vi "add.vi"(11 "LabVIEW Web Service Request":refnum<class "Web Request.lvclass">) -> ()   [LabVIEW 2014]
doc: "/lvwd-components-start/calc/add endpoint.\n\nExpects a JSON POST HTTP Request with a body containing a JSON object similar to the following:\n{ \"first\": \"5\", \"second\": \"6\" }\n\nA valid request returns a JSON object similar to the following:\n{\"sum\": 11}\n\nAn invalid request that is handelable returns HTTP Status Code 500 and a JSON object similar to:\n{\n \"message\": \"invalid parameters\",\n \"error\": {\n \"status\": true,\n \"code\": 5001,\n \"source\": \"notsoawesome.vi\",\n }\n}\n\nAn invalid request that cannot be handled MAY return an error code other than 200 and a response other than JSON (such as HTML, XML, etc)"
uses:
  <vilib>/wsapi/Web Request.lvclass
  Web Resources SubVIs/lvwd-components-start-calc.lvlib
  Utilities/lvwd-components-start-utilities.lvlib
panel:
  out "Error Out":errorcluster
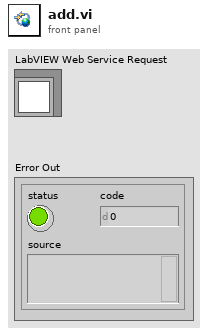
[diagram p1: front panel]
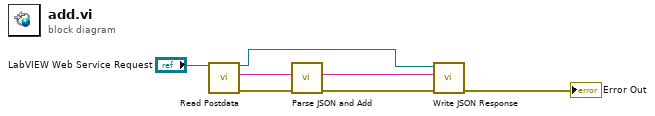
[diagram p0: block diagram]
diagram:
  n1 = call <vilib>:"Read Postdata.vi"("LabVIEW Web Service Request"="LabVIEW Web Service Request") -> ("LabVIEW Web Service Request out"=w1:refnum<class "Web Request.lvclass">, "postdata"=w5:string, "error out"=w6:errorcluster)  [unwired: 12 in]
  n2 = call "Parse JSON and Add.vi"("Error In"=w6, "JSON String In"=w5) -> ("Error Out"=w4:errorcluster, "JSON String Out"=w2:string)  [unwired: 8 in]
  n3 = call "Write JSON Response.vi"("Error In"=w4, "JSON Response"=w2, "LabVIEW Web Service Request In"=w1) -> ("Error Out"=→"Error Out":errorcluster)  [unwired: 7 in, 1 out]
